vi "e.gate HighSpeedPort Get Summary.vi"(8 "error in (no error)":errorcluster, 10 "Timeout (ms) [1000]":i32=1000, 11 "Configuration in":T1) -> (0 "error out":errorcluster, 3 "Configuration out":T1)   [LabVIEW 2016]
doc: "This VI reads the summray.sta file from an Gantner - Instruments e.series controller and saves it temporarily."
uses:
  e.gate Configuration.ctl
  e.gate Channel Data.ctl
  e.gate Data Type.ctl
  e.gate Protocol Type.ctl
  e.gate Module  Data.ctl
  e.gateHSP_DLLhandle.ctl
  e.gate HighSpeedPort Get File - Read FileData.vi
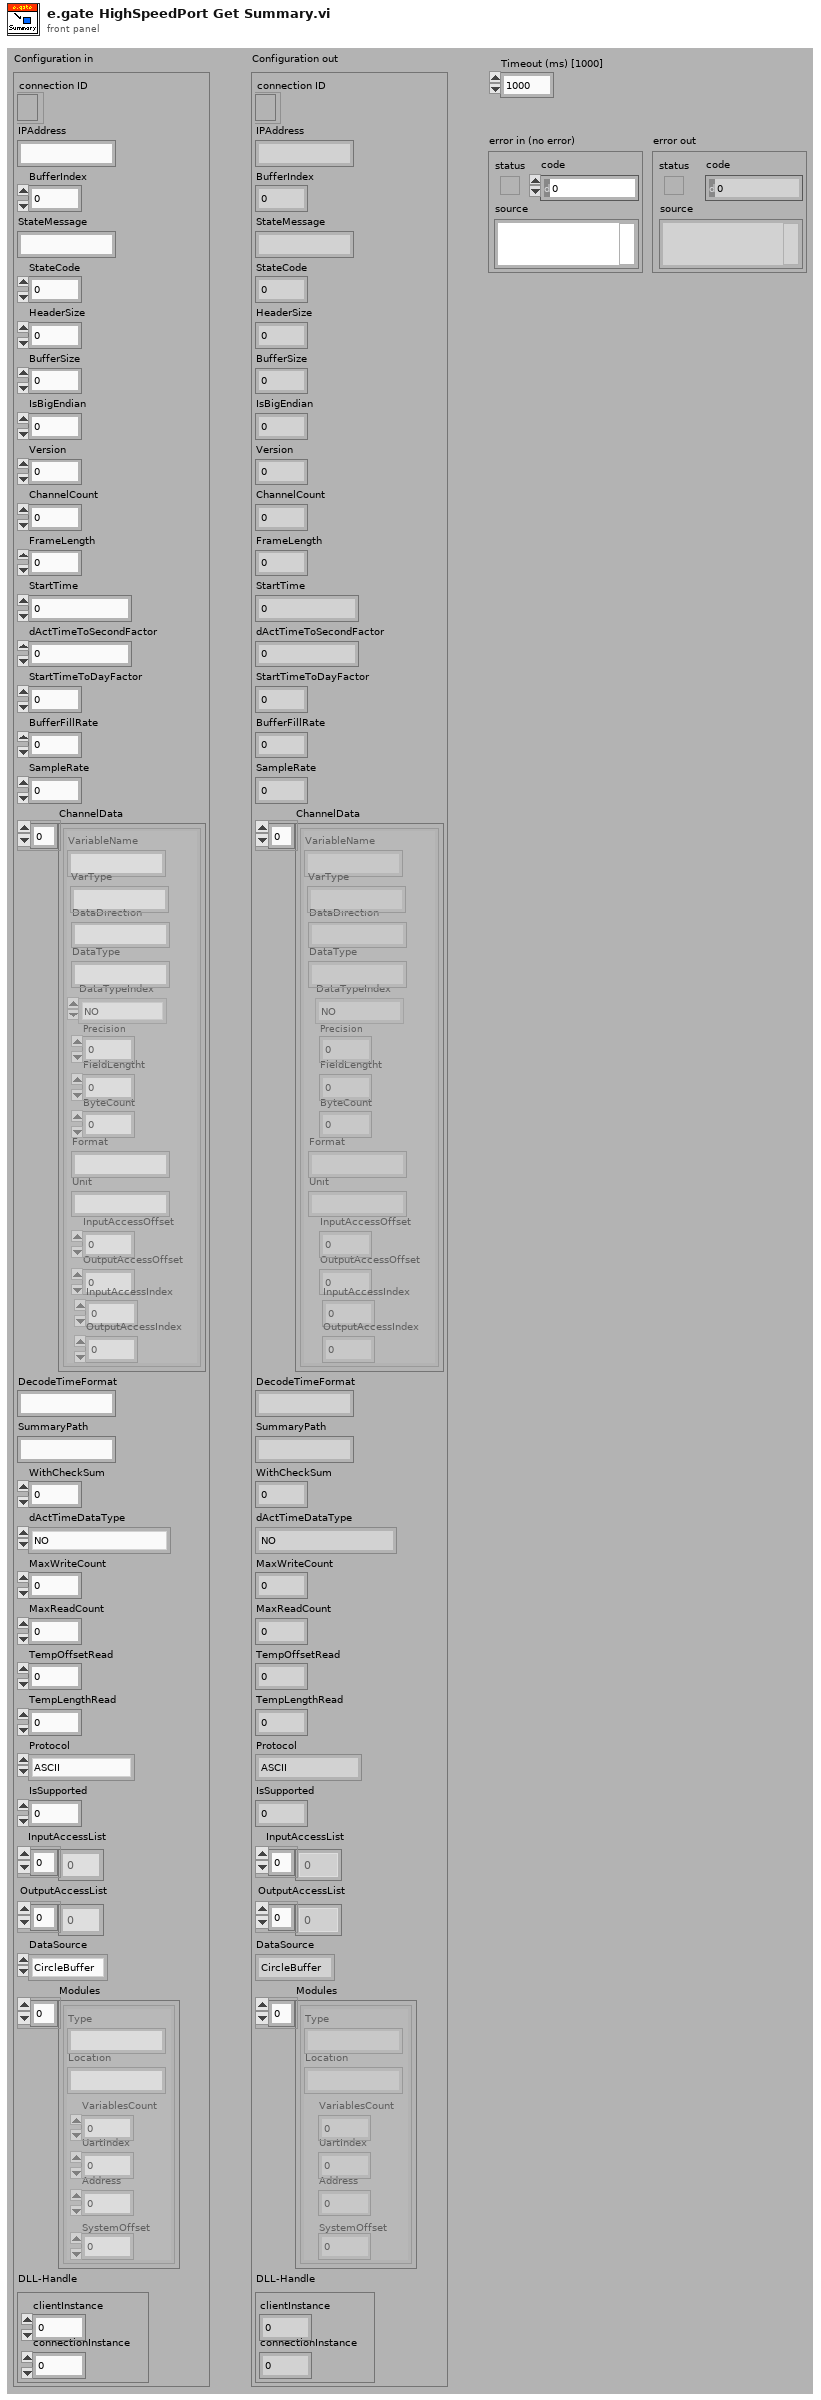
[diagram p1: front panel]
types:
  T1 = typedef "e.gate Configuration.ctl" = cluster{"connection ID":refnum<k5>, "IPAddress":string, "BufferIndex":i32, "StateMessage":string, "StateCode":i8, "HeaderSize":i32, "BufferSize":i32, "IsBigEndian":i32, "Version":i32, "ChannelCount":i32, "FrameLength":i32, "StartTime":dbl, "dActTimeToSecondFactor":dbl, "StartTimeToDayFactor":dbl, "BufferFillRate":dbl, "SampleRate":dbl, "ChannelData":T2[], "DecodeTimeFormat":string, "SummaryPath":string, "WithCheckSum":i32, "dActTimeDataType":T3, "MaxWriteCount":i32, "MaxReadCount":i32, "TempOffsetRead":i32, "TempLengthRead":i32, "Protocol":T4, "IsSupported":i32, "InputAccessList":i32[], "OutputAccessList":i32[], "DataSource":enum16{"CircleBuffer", "test.con Logger", "test.con Archive"}, "Modules":T5[], "DLL-Handle":T6}
  T2 = typedef "e.gate Channel Data.ctl" = cluster{"VariableName":string, "DataDirection":string, "DataType":string, "DataTypeIndex":T3, "Precision":i16, "FieldLengtht":i16, "ByteCount":i32, "Format":string, "Unit":string, "InputAccessOffset":i32, "OutputAccessOffset":i16, "InputAccessIndex":i16, "OutputAccessIndex":i16, "VarType":string}
  T3 = typedef "e.gate Data Type.ctl" = enum16{"NO", "BOOL", "SINT8", "USINT8", "SINT16", "USINT16", "SINT32", "USINT32", "FLOAT", "SET8", "SET16", "SET32", "DOUBLE", "SINT64", "USINT64", "SET64"}
  T4 = typedef "e.gate Protocol Type.ctl" = enum16{"ASCII", "HighspeedPort Online", "HighspeedPort Buffer", "eGateHighspeedPortDLL "}
  T5 = typedef "e.gate Module  Data.ctl" = cluster{"Type":string, "Location":string, "VariablesCount":i16, "UartIndex":i16, "Address":i16, "SystemOffset":i16}
  T6 = typedef "e.gateHSP_DLLhandle.ctl" = cluster{"clientInstance":i32, "connectionInstance":i32}
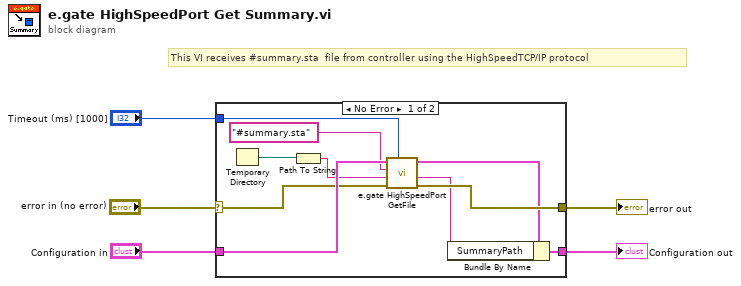
[diagram p0: block diagram]
diagram:
  # "This VI receives #summary.sta  file from controller using the HighSpeedTCP/IP protocol"
  n1 = case shown="No Error" "error in (no error)" {
    selector: "error in (no error)" -> [w9 w16]
    tunnel: [w15 w17] -> w4
    tunnel: "Configuration in" -> [w12 w17]
    tunnel: [w8 w16] -> w1
    tunnel: "Timeout (ms) [1000]" -> [w13 _]
    frame No Error {
      n2 = Temporary Directory() -> (w14:path)
      n3 = Path To String(path=w14) -> (string=w11:string)
      n4 = call-poly "e.gate HighSpeedPort GetFile.vi"("Timeout (ms) [1000]"=w13, "error in (no error)"=w9, "Destination Path"=w11, "File or relative Path"="#summary.sta", "Configuration in"=w12) -> ("error out"=w8:errorcluster, "Path Out"=w7:string, "Configuration out"=w6:T1)  [unwired: 4 out]
      n5 = Bundle By Name(cluster=w6, "SummaryPath"=w7) -> (w15:T1)
    }
    frame Error {
    }
  }
  "Configuration out" <- w4
  "error out" <- w1
